vi "Save.vi"(8 "error in":errorcluster, 10 "file path":path, 11 "SystemConfigRepo in":refnum<class "SystemConfigRepo.lvclass">) -> (0 "error out":errorcluster, 3 "SystemConfigRepo out":refnum<class "SystemConfigRepo.lvclass">)   [LabVIEW 2013, in "PL Framework Configuration Tool.lvlib" / "SystemConfigRepo.lvclass"]
uses:
  SystemConfigRepo.lvclass
  SystemConfigRepo.lvclass/SystemConfigRepo.ctl
  Framework Configuration Classes/platypus configuration/PLConfigurationSerializer.lvlib
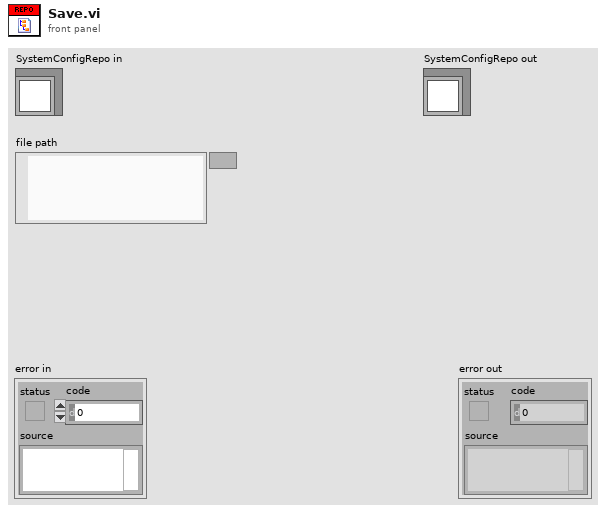
[diagram p1: front panel]
types:
  T1 = typedef "PLConfigurationSerializer.lvlib/systems cluster.ctl" = cluster{"System Configuration":refnum<class "PL_System Configuration.lvclass">, "targets":T2[]}
  T2 = typedef "PLConfigurationSerializer.lvlib/targets cluster.ctl" = cluster{"Target Configuration":refnum<class "PL_Target Configuration.lvclass">, "engines":T3[]}
  T3 = typedef "PLConfigurationSerializer.lvlib/engines cluster.ctl" = cluster{"engine configuration":refnum<class "engine configuration.lvclass">, "modules":refnum<class "TBM module configuration.lvclass">[]}
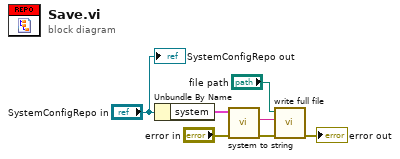
[diagram p0: block diagram]
diagram:
  n1 = Unbundle By Name("SystemConfigRepo in") -> ("system"=w3:T1)
  n2 = call "system to string.vi"("error in"="error in", "system"=w3) -> ("error out"=w1:errorcluster, "data"=w2:string)  [unwired: 8 in]
  n3 = call "write full file.vi"("error in"=w1, "data"=w2, "file path"="file path") -> ("error out"=→"error out":errorcluster)  [unwired: 8 in]
  "SystemConfigRepo out" <- "SystemConfigRepo in"
